vi "tt20_apply_settings.vi"(8 "error in (no error)":errorcluster, 10 "tt20_info":T1, 11 "tt20 in":refnum<class "tt20.lvclass">) -> (0 "error out":errorcluster, 3 "tt20 out":refnum<class "tt20.lvclass">)   [LabVIEW 2015, in "tt20.lvclass"]
uses:
  tt20.lvclass
  tt20_hardware_info_tdef.ctl
  tt20panel_class/tt20_acq_mode_tdef.ctl
  tt20.lvclass/tt20.ctl
  C:/Users/MX-Microscope/Documents/LabVIEW Data/lvoop_campus_2018/Detector_Class/Swabian/time_tagger_vis/TTCSharp32.dll
  time_tagger_vis/TTCSharp32.dll
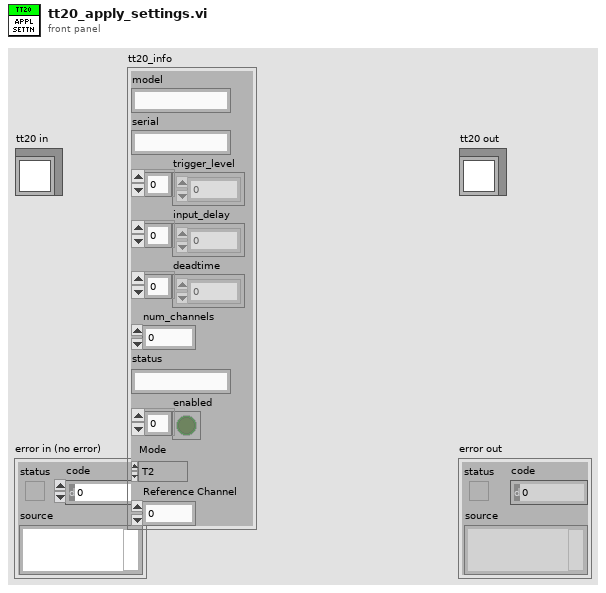
[diagram p1: front panel]
types:
  T1 = typedef "tt20_hardware_info_tdef.ctl" = cluster{"model":string, "serial":string, "trigger_level":dbl[], "input_delay":i64[], "deadtime":i64[], "num_channels":u32, "status":string, "enabled":bool[], "Mode":T2, "Reference Channel":u8}
  T2 = typedef "tt20_acq_mode_tdef.ctl" = enum16{"T2", "T3"}
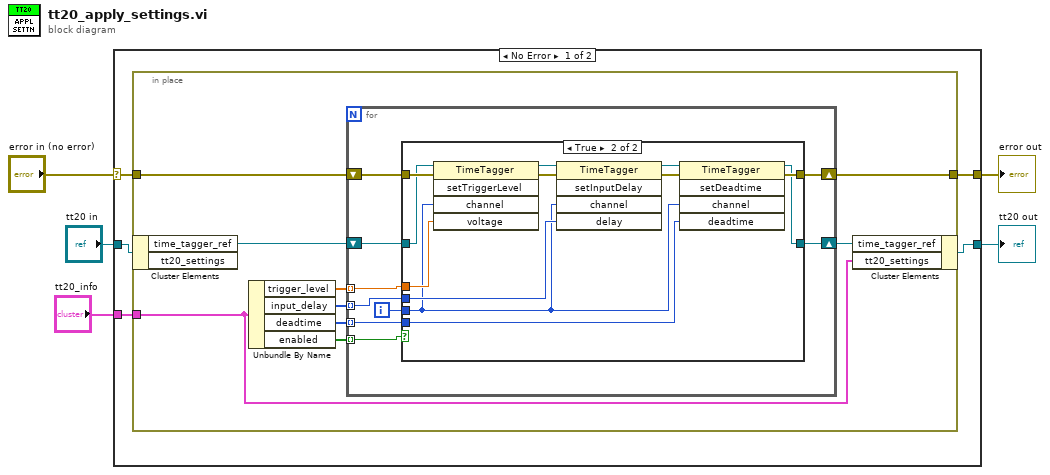
[diagram p0: block diagram]
diagram:
  n1 = case shown="No Error" "error in (no error)" {
    selector: "error in (no error)" -> [w8 w44]
    tunnel: [w7 w44] -> w4
    tunnel: [w6 w43] -> w2
    tunnel: "tt20 in" -> [w10 w43]
    tunnel: "tt20_info" -> [w9 _]
    frame No Error {
      n2 = in-place {
        in-place-border: w9 -> [w11]
        in-place-border: w8 -> [w18]
        in-place-border: [w14] -> w7
        n3 = in-place-cluster #1(w10) -> ("time_tagger_ref"=w17:refnum<k24>)  [unwired: 1 out]
        n4 = Unbundle By Name(w11) -> ("trigger_level"=w19:dbl[], "input_delay"=w16:i64[], "deadtime"=w15:i64[], "enabled"=w12:bool[])
        n5 = for {
          tunnel: w19 -> [w28] mode=indexing
          shift-right: [w21] -> w13
          shift-left: w17 -> [w26]
          tunnel: w16 -> [w25] mode=indexing
          tunnel: w15 -> [w23] mode=indexing
          shift-right: [w22] -> w14
          shift-left: w18 -> [w27]
          tunnel: w12 -> [w20] mode=indexing
          i -> [w24]
          n6 = case shown="True" w20 {
            tunnel: w28 -> [_ w42]
            tunnel: w27 -> [w30 w41]
            tunnel: w26 -> [w29 w40]
            tunnel: w25 -> [_ w38]
            tunnel: w24 -> [_ w34]
            tunnel: w23 -> [_ w33]
            tunnel: [w30 w32] -> w22
            tunnel: [w29 w31] -> w21
            frame False {
            }
            frame True {
              n7 = invoke class="TimeTagger" method="setTriggerLevel"(reference=w40, error in=w41, "channel"=w34, "voltage"=w42) -> (reference out=w39:refnum<k24>, error out=w37:errorcluster)  [unwired: 1 in, 3 out]
              n8 = invoke class="TimeTagger" method="setInputDelay"(reference=w39, error in=w37, "channel"=w34, "delay"=w38) -> (reference out=w36:refnum<k24>, error out=w35:errorcluster)  [unwired: 1 in, 3 out]
              n9 = invoke class="TimeTagger" method="setDeadtime"(reference=w36, error in=w35, "channel"=w34, "deadtime"=w33) -> (reference out=w31:refnum<k24>, error out=w32:errorcluster)  [unwired: 1 in, 3 out]
            }
          }
        }
        n10 = in-place-cluster #1("time_tagger_ref"=w13, "tt20_settings"=w11) -> (w6:refnum<class "tt20.lvclass">)
      }
    }
    frame Error {
    }
  }
  "error out" <- w4
  "tt20 out" <- w2
